vi "p11y1-3.vi"() -> ()   [LabVIEW 2020]
uses:
  Global 1.vi
panel:
  in  "stop":bool
  out "Juhuarv2":dbl
  out "Juhuarv1":dbl
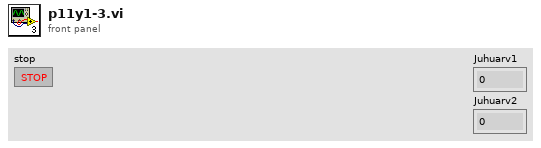
[diagram p1: front panel]
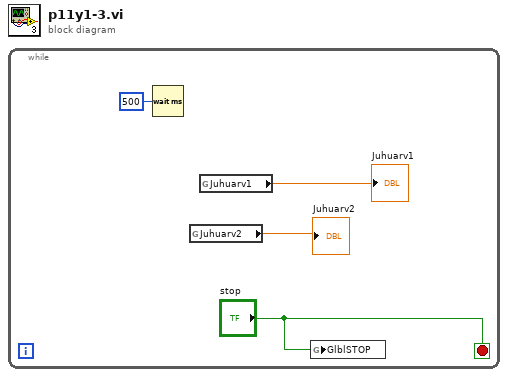
[diagram p0: block diagram]
diagram:
  n1 = while {
    stop <- "stop" stop-if-true
    n2 = Wait (ms)(milliseconds to wait=u32 500) -> ()  [unwired: 1 out]
    n3 = global read "Global 1.vi" "Juhuarv2"() -> (→"Juhuarv2":dbl)
    n4 = global read "Global 1.vi" "Juhuarv1"() -> (→"Juhuarv1":dbl)
    n5 = global write "Global 1.vi" "GlblSTOP"("stop") -> ()
  }
